vi "Wrapper For TypeSpecificAssert.vi"(8 "error in (no error)":errorcluster, 10 "U32 Array2":u32[](array[numeric]), 11 "U32 Array1":u32[](array[numeric])) -> (0 "error out":errorcluster)   [LabVIEW 2020]
uses:
  classes/Assert/Assert.lvclass
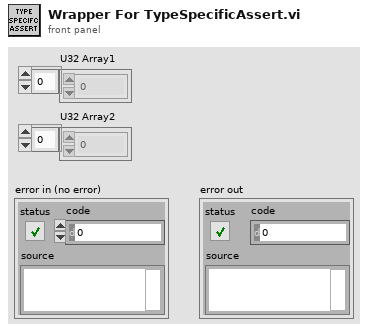
[diagram p1: front panel]
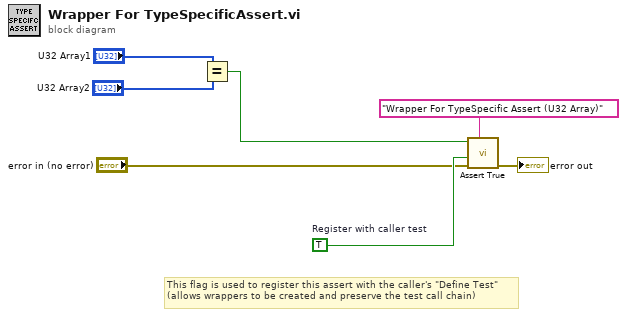
[diagram p0: block diagram]
diagram:
  w7 = TRUE  # Register with caller test
  # "This flag is used to register this assert with the caller's \"Define Test\"\n(allows wrappers to be created and preserve the test call chain)"
  n1 = Equal?(x="U32 Array1", y="U32 Array2") -> (x = y?=w1:bool)
  n2 = call "Assert True.vi"("Label"="Wrapper For TypeSpecific Assert (U32 Array)", "error in (no error)"="error in (no error)", "Register with caller test (F)"=w7, "True?"=w1) -> ("error out"=→"error out":errorcluster)  [unwired: 6 in, 1 out]
